vi "Create Channel Array.vi"(8 "error in":errorcluster, 10 "channel settings":T1[](array[typedef]), 11 "digital input mode in":refnum<class "Digital Input Mode.lvclass">) -> (0 "error out":errorcluster, 2 "channels":refnum<class "DI Channel.lvclass">[](array[class]), 3 "digital input mode out":refnum<class "Digital Input Mode.lvclass">)   [LabVIEW 2017, in "Scan Engine Scripting.lvlib" / "Digital Input Mode.lvclass"]
doc: "Instantiates and configures all channels for a module."
uses:
  Digital Input Mode.lvclass
  Controls/digital channel settings.ctl
  Channel Classes/DI Channel/DI Channel.lvclass
  Scan Engine Scripting.lvlib
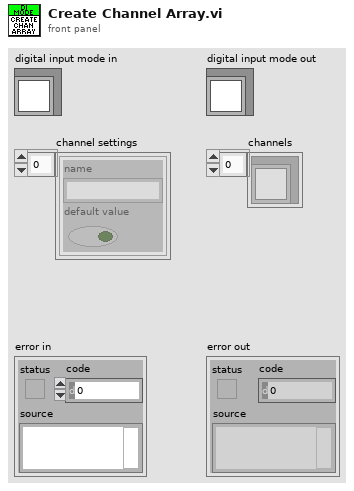
[diagram p1: front panel]
types:
  T1 = typedef "Scan Engine Scripting.lvlib/digital channel settings.ctl" = cluster{"name":string, "default value":bool}
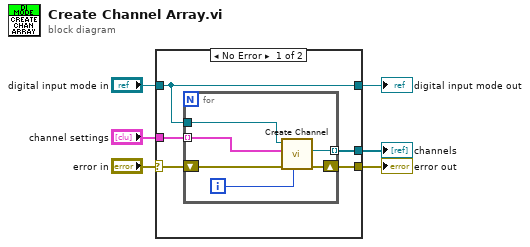
[diagram p0: block diagram]
diagram:
  n1 = case shown="No Error" "error in" {
    selector: "error in" -> [w10 w19]
    tunnel: [w7 w19] -> w5
    tunnel: [w9 w18] -> w3
    tunnel: "digital input mode in" -> [w9 w18]
    tunnel: "channel settings" -> [w11 _]
    tunnel: [w8 _] -> w1
    frame No Error {
      n2 = for {
        tunnel: w11 -> [w12] mode=indexing
        shift-right: [w16] -> w7
        shift-left: w10 -> [w17]
        tunnel: [w15] -> w8 mode=indexing
        tunnel: w9 -> [w14]
        i -> [w13]
        n3 = call "Create Channel.vi"("index"=w13, "error in"=w17, "settings"=w12, "digital input mode in"=w14) -> ("error out"=w16:errorcluster, "DI channel out"=w15:refnum<class "DI Channel.lvclass">)  [unwired: 5 in, 1 out]
      }
    }
    frame Error {
    }
  }
  "error out" <- w5
  "digital input mode out" <- w3
  "channels" <- w1
